vi "StripPathToPackageLevel_LV2015.vi"(8 "error in (no error)":errorcluster, 11 "Path in":path) -> (0 "error out":errorcluster, 3 "Path out":path)   [LabVIEW 2015]
panel:
  # "Connector Pane"
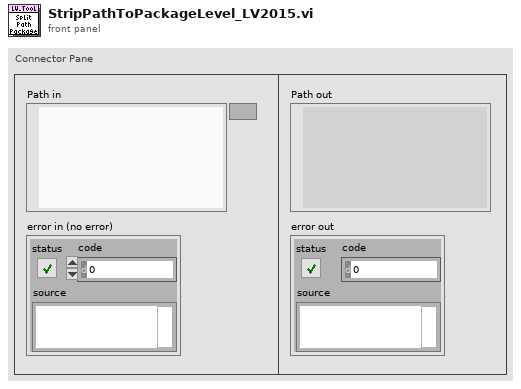
[diagram p1: front panel]
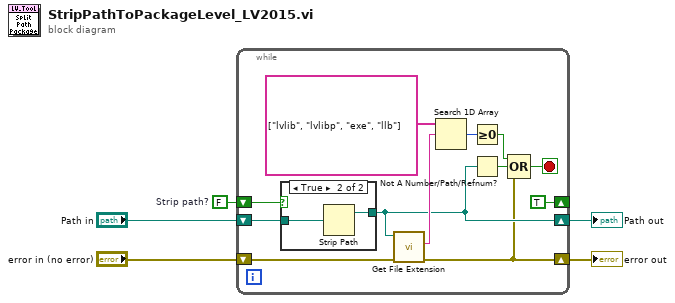
[diagram p0: block diagram]
diagram:
  w1 = FALSE  # Strip path?
  n1 = while {
    shift-right: [w10] -> w3
    shift-left: "Path in" -> [w17]
    shift-right: [w8] -> w5
    shift-left: "error in (no error)" -> [w16]
    shift-right: [TRUE ("Strip path?")] -> _
    shift-left: w1 -> [w7]
    stop <- w11 stop-if-true
    n2 = case shown="True" w7 {
      tunnel: w17 -> [w18 w20]
      tunnel: [w18 w19] -> w10
      frame False {
      }
      frame True {
        n3 = Strip Path(path=w20) -> (stripped path=w19:path)  [unwired: 1 out]
      }
    }
    n4 = call <vilib>:"Get File Extension.vi"("error in (no error)"=w16, "file"=w10) -> ("error out"=w8:errorcluster, "lowercase file extension"=w14:string)  [unwired: 5 in, 3 out]
    n5 = Search 1D Array(1D array=string[] ["lvlib", "lvlibp", "exe", "llb"] ("lowercase file extension"), element=w14) -> (index of element=w13:i32)  [unwired: 1 in]
    n6 = Greater Or Equal To 0?(x=w13) -> (x >= 0?=w12:bool)
    n7 = Not A Number/Path/Refnum?(number/path/refnum=w10) -> (NaN/Path/Refnum?=w9:bool)
    n8 = Compound Arithmetic op=OR(w12, w9, w8) -> (w11:bool)
  }
  "error out" <- w5
  "Path out" <- w3
